vi "Tektronix AFG 3000 Series Waveform Burst.vi"() -> ()   [LabVIEW 2015]
doc: "Demonstrates how to configure burst mode and trigger source.\n\nNote:\n\nFor external trigger source an external trigger input would be required."
uses:
  <instrlib>/Tektronix AFG 3000 Series/Tektronix AFG 3000 Series.lvlib
panel:
  in  "Burst Mode (0: Triggered)":u16(ring) items=["Triggered", "Gated"]
  in  "Channel (0: Channel 1)":u16(ring) items=["Channel 1", "Channel 2"]
  in  "Internal Trigger Rate (500)":dbl=500.0
  in  "Burst Count (5)":i32=5
  in  "VISA resource name":refnum<visa-resource-name>
  # "(c) 2006-2019 National Instruments.  ALL RIGHTS RESERVED."
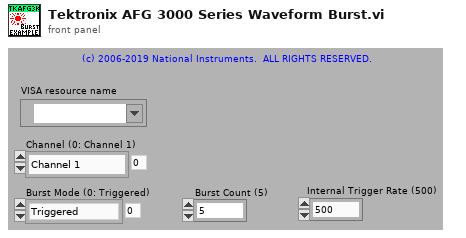
[diagram p1: front panel]
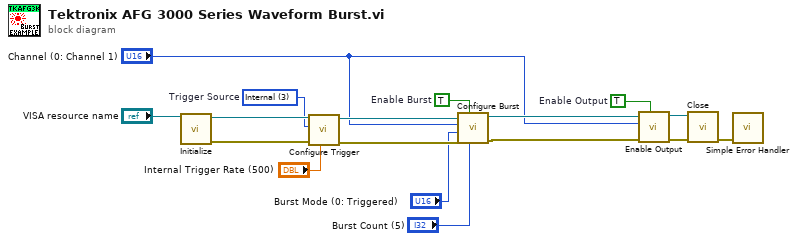
[diagram p0: block diagram]
diagram:
  w2 = u16 3 items=["Internal"=3, "External"=1]  # Trigger Source
  w7 = TRUE  # Enable Output
  w8 = TRUE  # Enable Burst
  n1 = call <instrlib>:"Initialize.vi"("VISA resource name"="VISA resource name") -> ("error out"=w3:errorcluster, "VISA resource name out"=w4:refnum<visa-resource-name>)  [unwired: 9 in]
  n2 = call <instrlib>:"Configure Trigger.vi"("Internal Trigger Rate (500)"="Internal Trigger Rate (500)", "error in (no error)"=w3, "Trigger Source (3:Internal)"=w2, "VISA resource name"=w4) -> ("error out"=w17:errorcluster, "VISA resource name out"=w16:refnum<visa-resource-name>)  [unwired: 6 in]
  n3 = call <instrlib>:"Configure Burst.vi"("Burst Count (5)"="Burst Count (5)", "Enable Burst (T: Enable)"=w8, "error in (no error)"=w17, "Burst Mode (0: Triggered)"="Burst Mode (0: Triggered)", "Channel (0: Channel 1)"="Channel (0: Channel 1)", "VISA resource name"=w16) -> ("error out"=w14:errorcluster, "VISA resource name out"=w15:refnum<visa-resource-name>)  [unwired: 4 in]
  n4 = call <instrlib>:"Enable Output.vi"("Enable Output (T: Enable)"=w7, "error in (no error)"=w14, "Channel (0: Channel 1)"="Channel (0: Channel 1)", "VISA resource name"=w15) -> ("error out"=w12:errorcluster, "VISA resource name out"=w13:refnum<visa-resource-name>)  [unwired: 6 in]
  n5 = call <instrlib>:"Close.vi"("error in (no error)"=w12, "VISA resource name"=w13) -> ("error out"=w11:errorcluster)  [unwired: 9 in]
  n6 = call <vilib>:"Simple Error Handler.vi"("error in (no error)"=w11) -> ()  [unwired: 4 in, 5 out]
